vi "Design FIR filter for N Waveforms.vi"(4 "optional FIR filter specifications":T2={"PB Gain"=3.0, "SB Gain"=60.0, "Scale"=TRUE, "Window"=enum."Flat Top"} {"SB Gain" format="%0.2f"; "PB Gain" format="%0.2f"}, 6 "FIR filter specifications":T3={"Topology"=enum."Off", "Type"=enum."Lowpass", "#Taps"=50, "Lower PB"=100.0, "Upper PB"=0.0, "Lower SB"=200.0, "Upper SB"=0.0} {"Lower SB" format="%0.2p"; "Upper SB" format="%0.2p"; "Lower PB" format="%0.2p"; "Upper PB" format="%0.2p"}, 7 "redesign filter":bool, 8 "error in":errorcluster, 11 "arrdt":dbl[](array[numeric]) format="%0.2f") -> (0 "error out":errorcluster, 1 "forward coefficients":dbl[](array[numeric]) format="%0.2f", 3 "filter information":T1 {"phase H(w)"."df" format="%0.2f"; "phase H(w)"."f0" format="%0.2f"; "phase H(w)"."Phase H(w)" format="%0.2f"; "magnitude H(w)"."df" format="%0.2f"; "magnitude H(w)"."f0" format="%0.2f"; "magnitude H(w)"."Mag H(w)" format="%0.2f"}, 5 "reset filters":bool)   [LabVIEW 2020, in "NI_MAPro.lvlib"]
uses:
  NI_MAPro.lvlib
  NI_MABase.lvlib
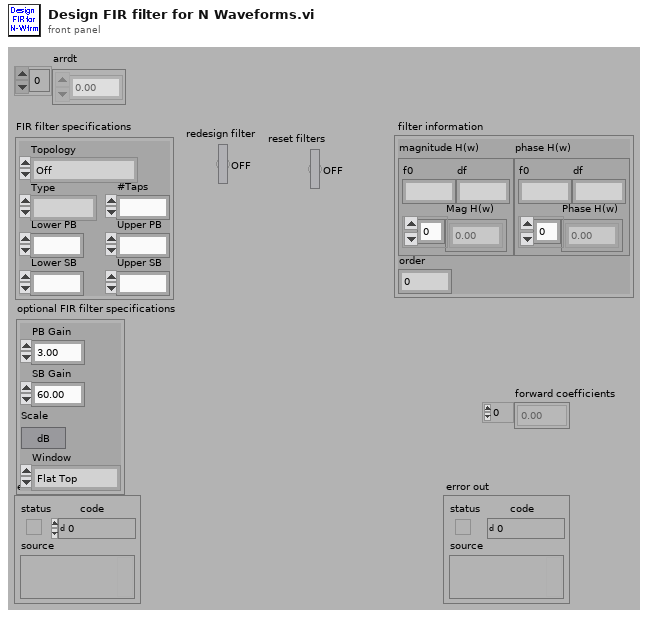
[diagram p1: front panel]
types:
  T1 = cluster{"magnitude H(w)":cluster{"f0":dbl, "df":dbl, "Mag H(w)":dbl[]}, "phase H(w)":cluster{"f0":dbl, "df":dbl, "Phase H(w)":dbl[]}, "order":i32}
  T2 = cluster{"PB Gain":dbl, "SB Gain":dbl, "Scale":bool, "Window":enum16{"None", "Hanning", "Hamming", "Triangular", "Blackman", "Exact Blackman", "Blackman-Harris", "Kaiser-Bessel", "Flat Top"}}
  T3 = cluster{"Topology":enum16{"Off", "FIR by Specification", "Equi-ripple FIR", "Windowed FIR"}, "Type":enum16{"Lowpass", "Highpass", "Bandpass", "Bandstop"}, "#Taps":i32, "Lower PB":dbl, "Upper PB":dbl, "Lower SB":dbl, "Upper SB":dbl}
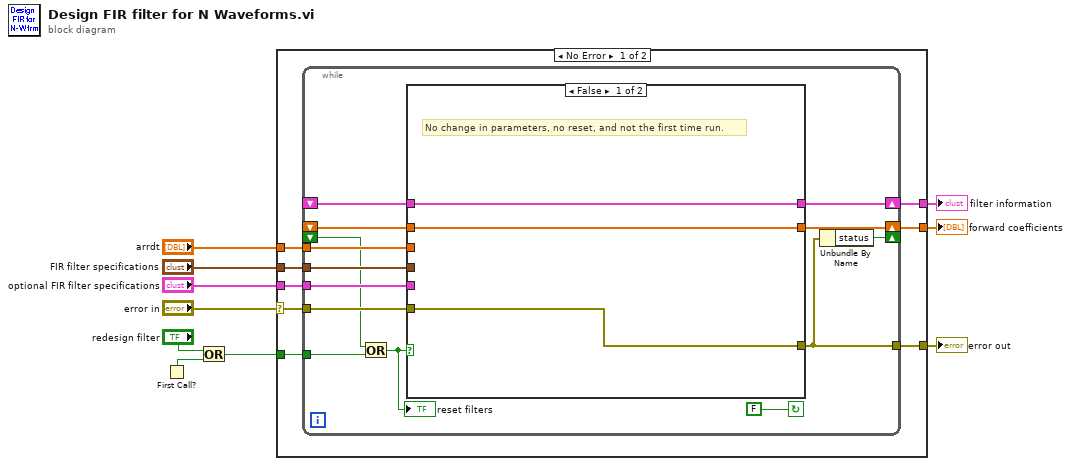
[diagram p0: block diagram]
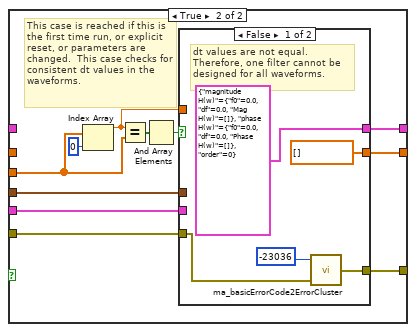
[diagram p2: hidden frame]
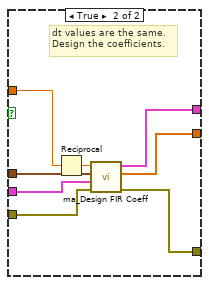
[diagram p3: hidden frame]
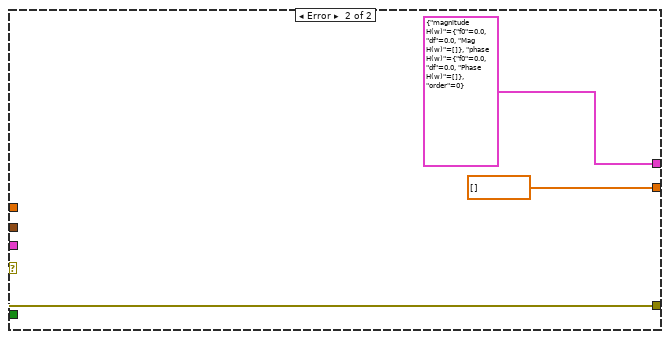
[diagram p4: hidden frame]
diagram:
  n1 = First Call?() -> (First Call?: T/F=w8:bool)
  n2 = Or(x="redesign filter", y=w8) -> (x .or. y?=w6:bool)
  n3 = case shown="No Error" "error in" {
    selector: "error in" -> [w17 w62]
    tunnel: [w18 w62] -> w10
    tunnel: w6 -> [w16 _]
    tunnel: "FIR filter specifications" -> [w15 _]
    tunnel: "optional FIR filter specifications" -> [w14 _]
    tunnel: [w13 dbl[] [] ("Forward Coefficients")] -> w3
    tunnel: [w12 T1 {"magnitude H(w)"={"f0"=0.0, "df"=0.0, "Mag H(w)"=[]}, "phase H(w)"={"f0"=0.0, "df"=0.0, "Phase H(w)"=[]}, "order"=0} ("Filter Information")] -> w2
    tunnel: "arrdt" -> [w11 _]
    frame No Error {
      n4 = while {
        tunnel: w11 -> [w25]
        tunnel: w14 -> [w28]
        tunnel: w15 -> [w26]
        tunnel: w17 -> [w24]
        tunnel: [w20] -> w18
        shift-left: _ -> [w29]
        shift-right: [w30] -> w12
        shift-left: _ -> [w32]
        shift-right: [w27] -> w13
        tunnel: w16 -> [w22]
        shift-right: [w19] -> _
        shift-left: _ -> [w23]
        stop <- FALSE continue-if-true
        n5 = Or(x=w23, y=w22) -> (x .or. y?=w21:bool)
        "reset filters" <- w21
        n6 = case shown="False" w21 {
          tunnel: w32 -> [w35 _]
          tunnel: [w34 w46] -> w30
          tunnel: w29 -> [w34 _]
          tunnel: [w35 w36] -> w27
          tunnel: [w33 w45] -> w20
          tunnel: w25 -> [_ w38]
          tunnel: w26 -> [_ w44]
          tunnel: w28 -> [_ w43]
          tunnel: w24 -> [w33 w42]
          frame False {
            # "No change in parameters, no reset, and not the first time run."
          }
          frame True {
            # "This case is reached if this is the first time run, or explicit reset, or parameters are changed.  This case checks for consistent dt values in the waveforms."
            n7 = Index Array(array=w38, index=0 ("Index")) -> (element=w37:dbl)
            n8 = Equal?(x=w37, y=w38) -> (x = y?=w40:bool[])
            n9 = And Array Elements(Boolean array=w40) -> (logical AND=w39:bool)
            n10 = case shown="False" w39 {
              tunnel: [T1 {"magnitude H(w)"={"f0"=0.0, "df"=0.0, "Mag H(w)"=[]}, "phase H(w)"={"f0"=0.0, "df"=0.0, "Phase H(w)"=[]}, "order"=0} ("Filter Information") w59] -> w46
              tunnel: [dbl[] [] ("Forward Coefficients") w58] -> w36
              tunnel: [w49 w57] -> w45
              tunnel: w44 -> [_ w55]
              tunnel: w43 -> [_ w54]
              tunnel: w42 -> [w47 w56]
              tunnel: w37 -> [_ w53]
              frame False {
                # "dt values are not equal.  \nTherefore, one filter cannot be \ndesigned for all waveforms."
                n11 = call "ma_basicErrorCode2ErrorCluster.vi"("error in (no error)"=w47, "Error Code"=-23036) -> ("error out"=w49:errorcluster)  [unwired: 1 in]
              }
              frame True {
                # "dt values are the same.  \nDesign the coefficients."
                n12 = Reciprocal(x=w53) -> (1/x=w52:dbl)
                n13 = call "ma_Design FIR Coeff.vi"("error in"=w56, "Optional FIR Filter Specifications"=w54, "FIR Filter Specifications"=w55, "Sampling Frequency"=w52) -> ("error out"=w57:errorcluster, "Forward Coefficients"=w58:dbl[], "Filter Information"=w59:T1)  [unwired: 5 in]
              }
            }
          }
        }
        n14 = Unbundle By Name(w20) -> ("status"=w19:bool)
      }
    }
    frame Error {
    }
  }
  "error out" <- w10
  "filter information" <- w2
  "forward coefficients" <- w3
